vi "Peak Density Compute Region to Region Edges.vi"(1 "All Regions":T1[][](array[typedef])) -> (0 "Edges":i32[][](array[numeric]))   [LabVIEW 2018, in "Video Cam Processor.lvclass"]
uses:
  Video Cam Processor.lvclass
  Private/Hull Point STYP.ctl
  0b8cf6e1-6ba8-4b16-9e8c-f60949ede83c.vi
  11663306-e135-4d54-a662-16468e77e369.vi
  cb8edd3f-1a2e-4d4d-9199-7cdf8b8af7c3.vi
  11663306-e135-4d54-a662-16468e77e369.vi/00458273-ef66-46b3-bacb-89d47f3423fa.vi
  cb8edd3f-1a2e-4d4d-9199-7cdf8b8af7c3.vi/74d1bef4-3758-4baa-894d-27f9f077a04d.vi
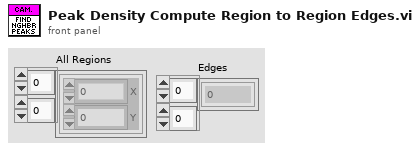
[diagram p1: front panel]
types:
  T1 = typedef "Video Cam Processor.lvclass/Hull Point STYP.ctl" = cluster{"X":i32, "Y":i32}
  T2 = typedef "Graham Scan Point.ctl" = cluster{"X":i32, "Y":i32}
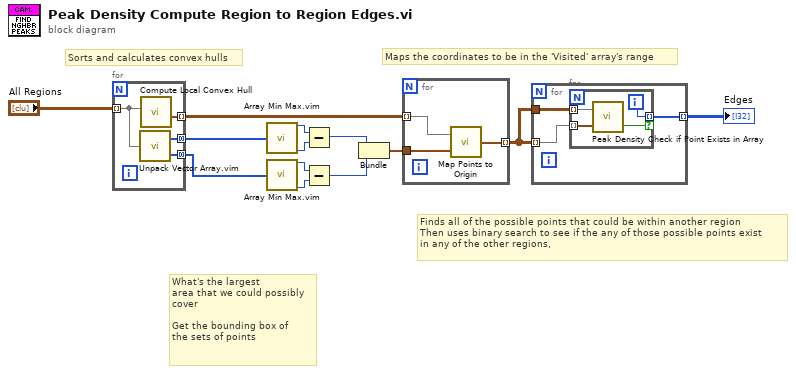
[diagram p0: block diagram]
diagram:
  # "Finds all of the possible points that could be within another region\nThen uses binary search to see if the any of those possible points exist\nin any of the other regions,"
  # "What's the largest\narea that we could possibly\ncover\n\nGet the bounding box of \nthe sets of points"
  # "Sorts and calculates convex hulls"
  # "Maps the coordinates to be in the 'Visited' array's range"
  n1 = for {
    tunnel: "All Regions" -> [w15] mode=indexing
    tunnel: [w14] -> w6 mode=indexing
    tunnel: [w17] -> w12 mode=concatenating
    tunnel: [w16] -> w11 mode=concatenating
    n2 = call "Unpack Vector Array.vim"("Vector Array"=w15) -> ("Y Array"=w16:i32[], "X Array"=w17:i32[])  [unwired: 2 in]
    n3 = call "Compute Local Convex Hull.vi"("Included Points"=w15) -> ("Convex Hull"=w14:T2[])  [unwired: 5 in, 1 out]
  }
  n4 = call "Array Min Max.vim"("Array"=w12) -> ("Max"=w10:i32, "Min"=w9:i32)  [unwired: 13 in]
  n5 = call "Array Min Max.vim"("Array"=w11) -> ("Max"=w8:i32, "Min"=w7:i32)  [unwired: 13 in]
  n6 = Subtract(x=w10, y=w9) -> (x-y=w4:i32)
  n7 = Subtract(x=w8, y=w7) -> (x-y=w5:i32)
  n8 = Bundle(w4, w5) -> (w3:cluster{i32, i32})  [unwired: 1 in]
  n9 = for {
    tunnel: w3 -> [w19]
    tunnel: w6 -> [w20] mode=indexing
    tunnel: [w18] -> w2 mode=indexing
    n10 = call "Map Points to Origin.vi"("New Origin"=w19, "Points"=w20) -> ("Mapped Points"=w18:T2[])
  }
  n11 = for {
    tunnel: w2 -> [w22] mode=indexing
    tunnel: w2 -> [w23]
    tunnel: [w21] -> w1 mode=indexing
    n12 = for {
      tunnel: w23 -> [w27] mode=indexing
      tunnel: w22 -> [w26] mode=indexing
      tunnel: [w25] -> w21 mode=indexing if=w24
      i -> [w25]
      n13 = call "Peak Density Check if Point Exists in Array.vi"("Point"=w26, "Array"=w27) -> ("Exists?"=w24:bool)  [unwired: 1 out]
    }
  }
  "Edges" <- w1
